vi "TimeLapse ini AVI & header file.vi"(8 "error in (no error)":errorcluster) -> (0 "error out":errorcluster)   [LabVIEW 2013]
uses:
  Typedefs/Channel Selector.ctl
  User Interface/Visualisation/Functional Imaging Viewer/SubVIs/Experiment header interface/Typedefs/Header file type enum.ctl
  Global Variables/General Globals.vi
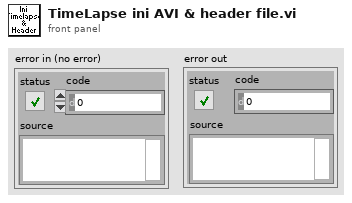
[diagram p1: front panel]
types:
  T1 = typedef "Header file type enum.ctl" = enum16{"All parameters", "Params for funct acq w ROI or mscn", "Params for funct acq w rectangles", "Live imaging header parameters", "AOL Parameters"}
  T2 = typedef "Channel Selector.ctl" = enum16{"Red Channel", "Green Channel", "Blended"}
  T3 = typedef "AOL_Globals.ctl" = cluster{"Imaging Protocol":T4, "Number of POI":u16, "Number of Miniscans":u16, "Number of Trials":u16, "Number of Cycles ":u64, "# Averaged Frames":u16, "Laser power (%)":u8, "Pockels":dbl, "Acquisition Length (sec)":dbl, "Fill time (us)":dbl, "POI Dwell time (us)":dbl, "Miniscan Dwell time per pixel (us)":dbl, "PMT 1":dbl, "PMT 2":dbl, "Back Apperture":dbl, "Frame Size":T5, "Center Frequency":dbl, "Field of View":dbl, "DwellTime (us)":dbl, "Wavelength (nm)":dbl, "Zoom":dbl, "AOL Z":dbl, "AOL Mode":T6, "GridXY":dbl, "GridZ":dbl, "TriggerPeriod (sec)":dbl, "Number of Pixels in Miniscan":u16, "Experiment folder path":path, "X centre":dbl, "Y centre":dbl, "Angle (degrees)":dbl, "Plane Mode":T7, "Threshold":u16[], "Regenerate Chirps":bool, "Rectangle ROI length (pixels)":u16, "Rectangle ROI height (pixels)":u16, "AOD fill":u16, "Samples Wait after Trigger":u16, "StartUp Delay":i32, "Slip Cycle":u32, "Add Cycle":bool}
  T4 = typedef "Imaging Protocols enum.ctl" = enum16{"AOL Z-Stack", "Motor Z Stack", "Functional Acquisition", "Single Plane Acquisition", "Volume Acquisition", "Live Imaging", "Live Plane Imaging", "Live Volume Imaging"}
  T5 = typedef "Frame Size.ctl" = u16
  T6 = typedef "AOL modes.ctl" = enum16{"Raster", "Structural", "Pointing", "Mini Scan", "Alignment"}
  T7 = typedef "Plane Mode.ctl" = u16
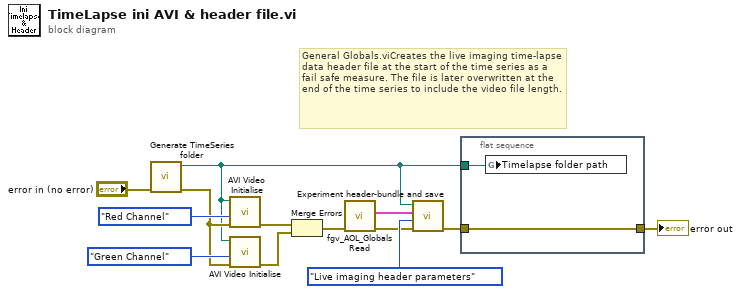
[diagram p0: block diagram]
diagram:
  # "General Globals.viCreates the live imaging time-lapse data header file at the start of the time series as a fail safe measure. The file is later overwritten at the end of the time series to include the video file length."
  n1 = call "Generate TimeSeries folder.vi"("error in (no error)"="error in (no error)") -> ("error out"=w3:errorcluster, "Timelapse folder path"=w2:path)  [unwired: 9 in]
  n2 = call "AVI Video Initialise.vi"("error in (no error)"=w3, "Channel"=Channel_Selector."Red Channel", "Timelapse folder path"=w2) -> ("error out"=w12:errorcluster)  [unwired: 8 in]
  n3 = call "AVI Video Initialise.vi"("error in (no error)"=w3, "Channel"=Channel_Selector."Green Channel", "Timelapse folder path"=w2) -> ("error out"=w13:errorcluster)  [unwired: 8 in]
  n4 = Merge Errors(w12, w13) -> (w5:errorcluster)
  n5 = call "fgv_AOL_Globals Read.vi"("error in (no error)"=w5) -> ("error out"=w4:errorcluster, "AOL_Globals"=w1:T3)  [unwired: 8 in, 1 out]
  n6 = call "Experiment header-bundle and save.vi"("error in (no error)"=w4, "Header file type"=Header_file_type_enum."Live imaging header parameters", "AOL_Globals"=w1, "Experiment data folder path"=w2) -> ("error out"=w7:errorcluster)  [unwired: 7 in]
  n7 = flat-sequence {
    tunnel: w7 -> [w15]
    tunnel: [w15] -> w6
    tunnel: w2 -> [w14]
    frame #0 {
      n8 = global write "General Globals.vi" "Timelapse folder path"(w14) -> ()
    }
  }
  "error out" <- w6
